vi "Gen_Test_Single_Cell_2.vi"() -> ()   [LabVIEW 2020]
panel:
  in  "Output Safety":T1
  in  "filepath":path
  in  "Batteryname":string
  in  "Starting Cycle":i32
  out "PS error out":errorcluster
  out "PS VIS resource name out":refnum<visa-resource-name>
  in  "Charge Current Cutoff":dbl
  in  "Charge Current Setpoint 2":dbl format="%#.6g"
  in  "charge Voltage Setpoint  2":dbl format="%#.6g"
  in  "Wait time":dbl
  in  "Discharge Current Cutoff":dbl
  in  "Discharge Current Setpoint":dbl format="%#.6g"
  in  "Discharge Voltage Setpoint":dbl format="%#.6g"
  in  "NHR VISA":refnum<visa-resource-name>
  in  "NHR error in":errorcluster
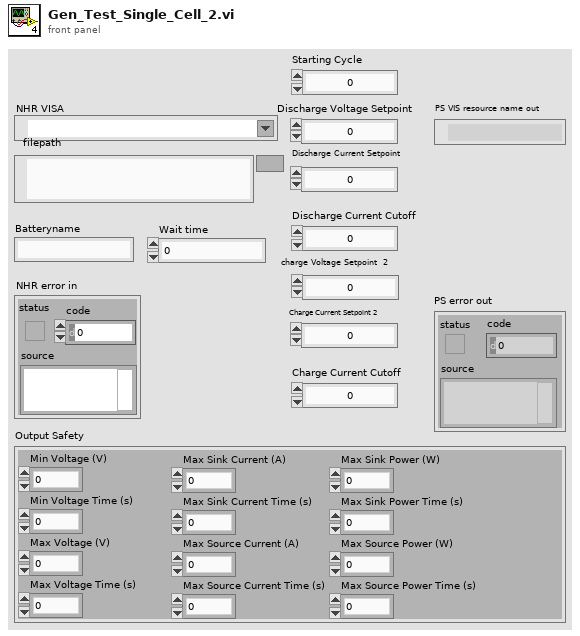
[diagram p1: front panel]
types:
  T1 = cluster{"Min Voltage (V)":dbl, "Min Voltage Time (s)":dbl, "Max Voltage (V)":dbl, "Max Voltage Time (s)":dbl, "Max Sink Current (A)":dbl, "Max Sink Current Time (s)":dbl, "Max Source Current (A)":dbl, "Max Source Current Time (s)":dbl, "Max Sink Power (W)":dbl, "Max Sink Power Time (s)":dbl, "Max Source Power (W)":dbl, "Max Source Power Time (s)":dbl}
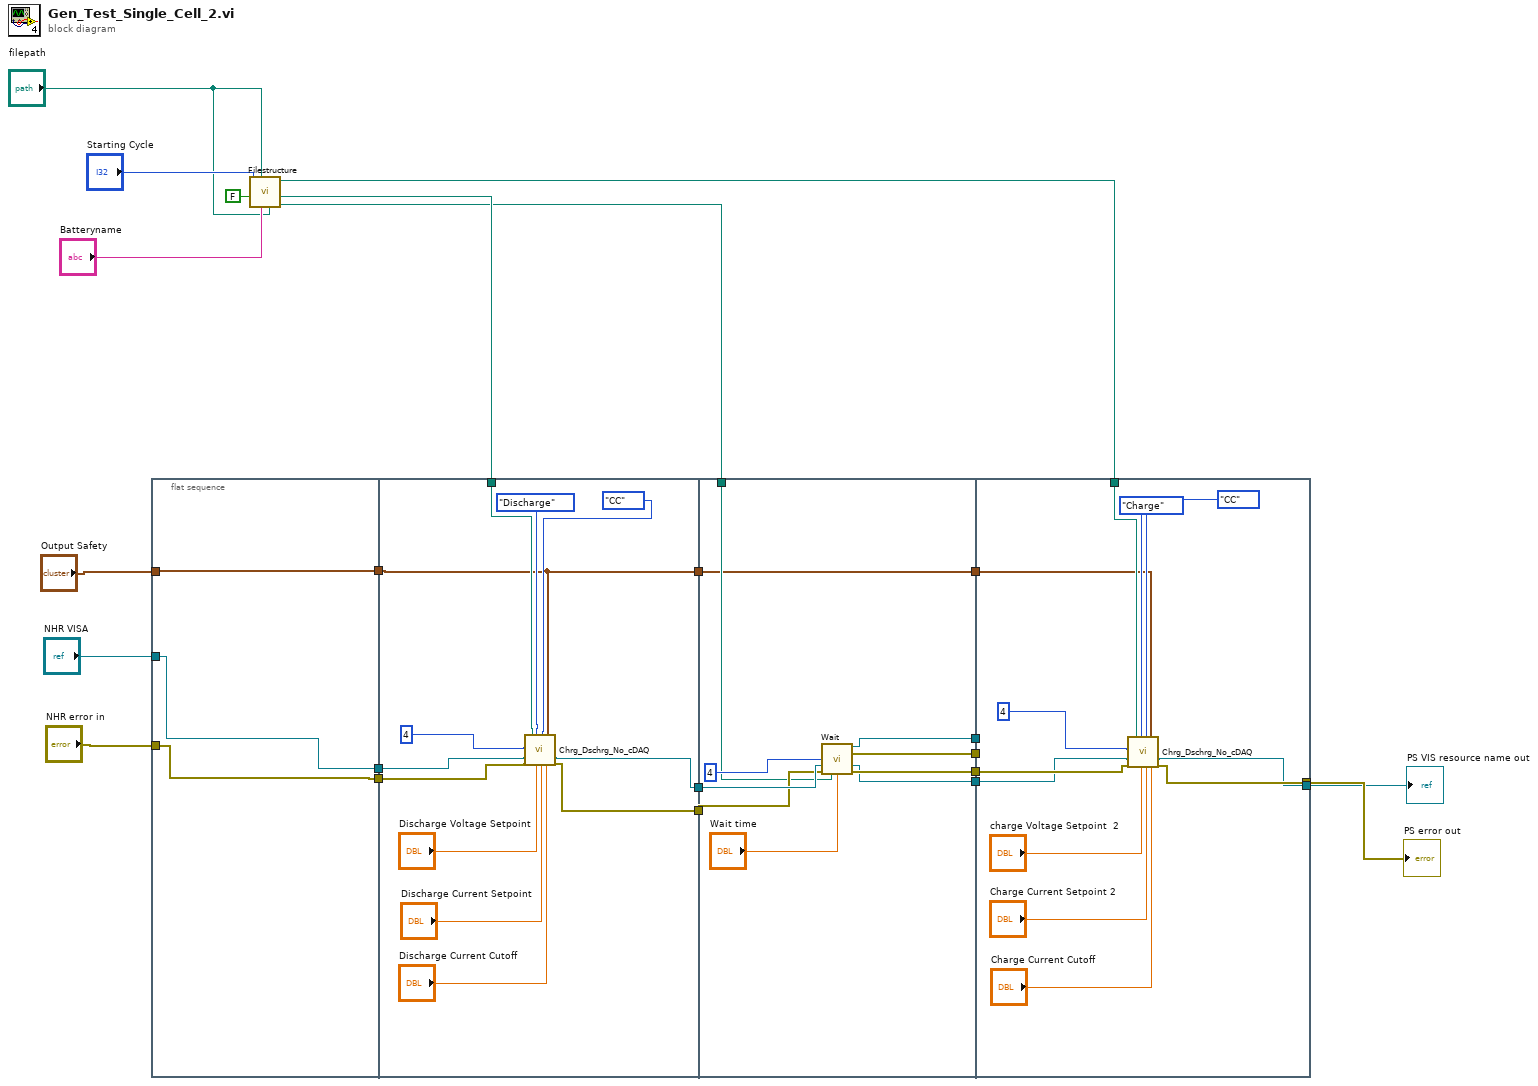
[diagram p0: block diagram]
diagram:
  n1 = flat-sequence {
    tunnel: "NHR error in" -> [w25]
    tunnel: "NHR VISA" -> [w26]
    tunnel: [w26] -> w21
    tunnel: [w25] -> w20
    tunnel: "Output Safety" -> [w24]
    tunnel: [w24] -> w4
    tunnel: w21 -> [w32]
    tunnel: w20 -> [w33]
    tunnel: [w38] -> w19
    tunnel: [w37] -> w18
    tunnel: w8 -> [w30]
    tunnel: w4 -> [w27]
    tunnel: [w27] -> w3
    tunnel: w19 -> [w47]
    tunnel: w18 -> [w46]
    tunnel: [w39] -> w17
    tunnel: [w44] -> w16
    tunnel: [w43] -> w15
    tunnel: [w42] -> w14
    tunnel: w7 -> [w41]
    tunnel: w3 -> [w40]
    tunnel: [w40] -> w2
    tunnel: w17 -> [_]
    tunnel: w16 -> [_]
    tunnel: w15 -> [w57]
    tunnel: w14 -> [w56]
    tunnel: [w50] -> w13
    tunnel: [w49] -> w12
    tunnel: w6 -> [w54]
    tunnel: w2 -> [w51]
    frame #0 {
    }
    frame #1 {
      n2 = call "Chrg_Dschrg_No_cDAQ.vi"("Thermocouple"=4 ("#DAQ outputs (1-13)"), "PS VISA in"=w32, "PS error in"=w33, "DischargeCyclePath"=w30, "Charge/discharge"=enum8{"Charge", "Discharge"}."Discharge", "Charge/Discharge Voltage Setpoint"="Discharge Voltage Setpoint", "CC or CCCV"=enum16{"CC", "CCCV"}."CC", "Current Setpoint"="Discharge Current Setpoint", "Output Safety"=w27, "Current Cutoff"="Discharge Current Cutoff") -> ("PS VIS resource name out"=w38:refnum<visa-resource-name>, "PS error out"=w37:errorcluster)  [unwired: 8 in]
    }
    frame #2 {
      n3 = call "Wait.vi"("#DAQ outputs (1-13)"=4, "PS VISA in"=w47, "PS error in"=w46, "Wait Filepath"=w41, "Wait time"="Wait time") -> ("data task out"=w39:refnum<k21>, "data task error out"=w44:errorcluster, "PS Visa Out"=w42:refnum<visa-resource-name>, "PS error out"=w43:errorcluster)  [unwired: 7 in]
    }
    frame #3 {
      n4 = call "Chrg_Dschrg_No_cDAQ.vi"("Thermocouple"=4 ("#DAQ outputs (1-13)"), "PS VISA in"=w56, "PS error in"=w57, "DischargeCyclePath"=w54, "Charge/discharge"=enum8{"Charge", "Discharge"}."Charge", "Charge/Discharge Voltage Setpoint"="charge Voltage Setpoint  2", "CC or CCCV"=enum16{"CC", "CCCV"}."CC", "Current Setpoint"="Charge Current Setpoint 2", "Output Safety"=w51, "Current Cutoff"="Charge Current Cutoff") -> ("PS VIS resource name out"=w49:refnum<visa-resource-name>, "PS error out"=w50:errorcluster)  [unwired: 8 in]
    }
  }
  n5 = call "Filestructure.vi"("Discharge filepath"="filepath", "Batteryname"="Batteryname", "Charge filepath"="filepath", "In for loop"=FALSE, "Starting Cycle"="Starting Cycle") -> ("DischargeWaitPath"=w7:path, "DischargeCyclePath"=w8:path, "ChargeCyclePath"=w6:path)  [unwired: 2 in, 2 out]
  "PS error out" <- w13
  "PS VIS resource name out" <- w12
